vi "FTW-TransferClient-PostEvent-Status.vi"(4 "Error Message":string, 5 "Timestamp":u32, 6 "Error?":bool, 7 "Initial Timestamp":u32, 8 "Cancelled?":bool, 9 "Local Filepath":path, 10 "Remote URI":string, 11 "Transfer Status Event":refnum<user-event>) -> ()   [LabVIEW 2012, in "FTW-TransferClient.lvclass"]
uses:
  FTW-TransferClient.lvclass
  FTW-TransferClient-TransferStatus.ctl
panel:
  # "Inputs"
  # "Outputs"
  # "No Outputs - this VI\nis fire and forget"
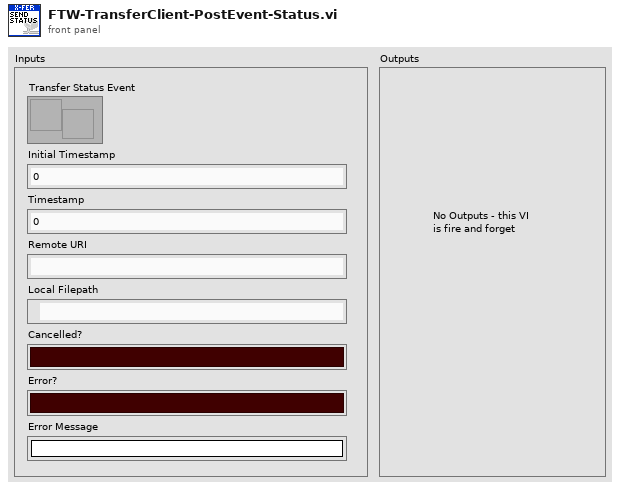
[diagram p1: front panel]
types:
  T1 = typedef "FTW-TransferClient-TransferStatus.ctl" = cluster{"Remote URI":string, "Local Filepath":path, "Cancelled?":bool, "Error?":bool, "Error Message":string, "Time Elapsed":u32}
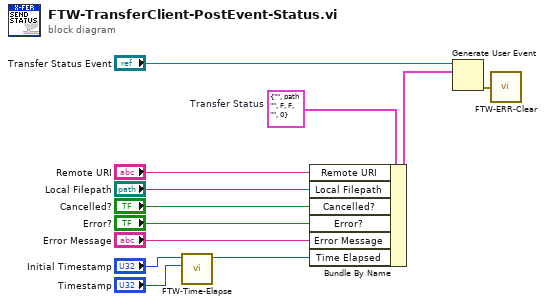
[diagram p0: block diagram]
diagram:
  w5 = T1 {"Remote URI"="", "Local Filepath"=path "", "Cancelled?"=FALSE, "Error?"=FALSE, "Error Message"="", "Time Elapsed"=0}  # Transfer Status
  n1 = call "FTW-Time-Elapse.vi"("End Time"="Timestamp", "Initial Time"="Initial Timestamp") -> ("Elapsed msec"=w1:u32)  [unwired: 8 in, 1 out]
  n2 = Bundle By Name(cluster=w5, "Remote URI"="Remote URI", "Local Filepath"="Local Filepath", "Cancelled?"="Cancelled?", "Error?"="Error?", "Error Message"="Error Message", "Time Elapsed"=w1) -> (w12:T1)
  n3 = Generate User Event(user event="Transfer Status Event", event data cluster=w12) -> (error out=w6:errorcluster)  [unwired: 1 in, 1 out]
  n4 = call "FTW-ERR-Clear.vi"("error to snuff"=w6) -> ()  [unwired: 1 out]
